vi "Append Block Diagram Image.vi"(0 "PDF Report IN":refnum<class "PDF Report Class.lvclass">, 1 "Image size":T1={"Maximum Width"=-1, "Maximum Height"=-1}, 2 "Scale (%)":sgl=100.0, 3 "Border":T2={"Show?"=FALSE, "Thickness (point)"=0.5, "Color"=0}, 5 "VI reference":refnum<vi>, 11 "error in (no error)":errorcluster, 12 "Caption":string, 14 "Position and indentation":T3={"Alignment"=enum."Center", "X "=0.0, "Y"=0.0, "Indentation"=0.0}) -> (4 "PDF Report OUT":refnum<class "PDF Report Class.lvclass">, 15 "error out":errorcluster)   [LabVIEW 2020, in "Exaprom PDF.lvlib"]
doc: "Creates an image of the block diagram of the VI you specify in <B>VI reference</B> and appends it to a PDF report. <B>Not Available in Run-Time </B>.\n\n<B>FRANÇAIS</B>\nCréation de l'image du \"block diagram\" que vous avez spécifié par <B>VI reference</B> et ajout au rapport PDF. <B>Ce VI fonctionne uniquement en mode développement</B>.\n\nVersion 1.0\nDeveloped by Jean-Marc Simard\nCopyright © 2010, Exaprom Inc.\nAll rights reserved.\nLicense: BSD\n\nWith iTextSharp 4.1.6 (http://itextsharp.sourceforge.net)\nunder Mozilla Public License Version 1.1\n(http://www.mozilla.org/MPL/MPL-1.1.html)"
uses:
  <userlib>/labview-PDF-writer-master/Exaprom PDF.lvlib
  <userlib>/labview-PDF-writer-master/LV Class/PDF Report Class/PDF Report Class.lvclass
  <userlib>/labview-PDF-writer-master/Controls/Image Controls/Image alignment and position.ctl
  <userlib>/labview-PDF-writer-master/Controls/Image Controls/Image aligment.ctl
  <userlib>/labview-PDF-writer-master/Controls/Image Controls/Image border.ctl
  <userlib>/labview-PDF-writer-master/Controls/Image Controls/Image Size Block Diagram.ctl
  <userlib>/labview-PDF-writer-master/Controls/Font Controls/Font complete cluster.ctl
  <userlib>/labview-PDF-writer-master/Controls/Font Controls/Font size.ctl
  <userlib>/labview-PDF-writer-master/Controls/Font Controls/Font color.ctl
  <userlib>/labview-PDF-writer-master/Controls/Font Controls/Type and encoding.ctl
  <userlib>/labview-PDF-writer-master/Controls/Text Controls/Unicode/Type and run direction.ctl
  C:/Program Files (x86)/National Instruments/LabVIEW 2020/user.lib/labview-PDF-writer-master/DLL/itextsharp.dll
  DLL/itextsharp.dll
panel:
  out "Size (points)":cluster{"TotalHeight":sgl, "TotalWidth":sgl}
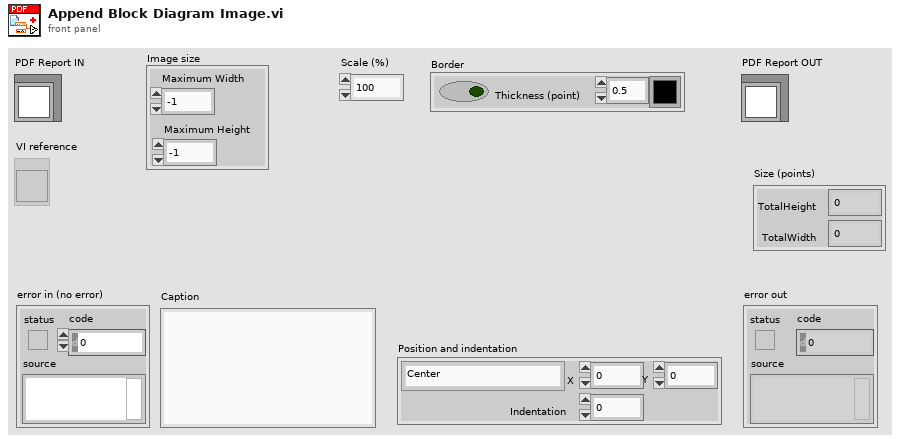
[diagram p1: front panel]
types:
  T1 = typedef "Exaprom PDF.lvlib/Image Size Block Diagram.ctl" = cluster{"Maximum Width":i32, "Maximum Height":i32}
  T2 = typedef "Exaprom PDF.lvlib/Image border.ctl" = cluster{"Show?":bool, "Thickness (point)":sgl, "Color":u32}
  T3 = typedef "Exaprom PDF.lvlib/Image alignment and position.ctl" = cluster{"Alignment":T4, "X ":sgl, "Y":sgl, "Indentation":sgl}
  T4 = typedef "Exaprom PDF.lvlib/Image aligment.ctl" = enum16{"Absolute (X,Y)", "Left", "Center", "Right", "Left (textwrap)", "Right (textwrap)"}
  T5 = typedef "Exaprom PDF.lvlib/Font complete cluster.ctl" = cluster{"Name":string, "Size":T6, "Color":T7, "Style":cluster{"Bold":bool, "Italic":bool, "Underline":bool, "Strikeout":bool}, "Type":T8}
  T6 = typedef "Exaprom PDF.lvlib/Font size.ctl" = sgl
  T7 = typedef "Exaprom PDF.lvlib/Font color.ctl" = u32
  T8 = typedef "Exaprom PDF.lvlib/Type and encoding.ctl" = cluster{"Type&direction":T9, "Embedded":bool, "Encoding":string}
  T9 = typedef "Exaprom PDF.lvlib/Type and run direction.ctl" = enum16{"Select", "ASCII", "UTF-16", "UTF-16 (default)", "UTF-16 (LTR)", "UTF-16 (RTL)"}
  T10 = enum32{"invalid app kind", "Development System", "Run Time System", "Student Edition", "Embedded LabVIEW", "Evaluation", "Custom"}
  T11 = typedef "imagedata.ctl" = cluster{"image type":i32, "image depth":i32, "image":u8[], "mask":u8[], "colors":u32[], "Rectangle":cluster{"left":i16, "top":i16, "right":i16, "bottom":i16}}
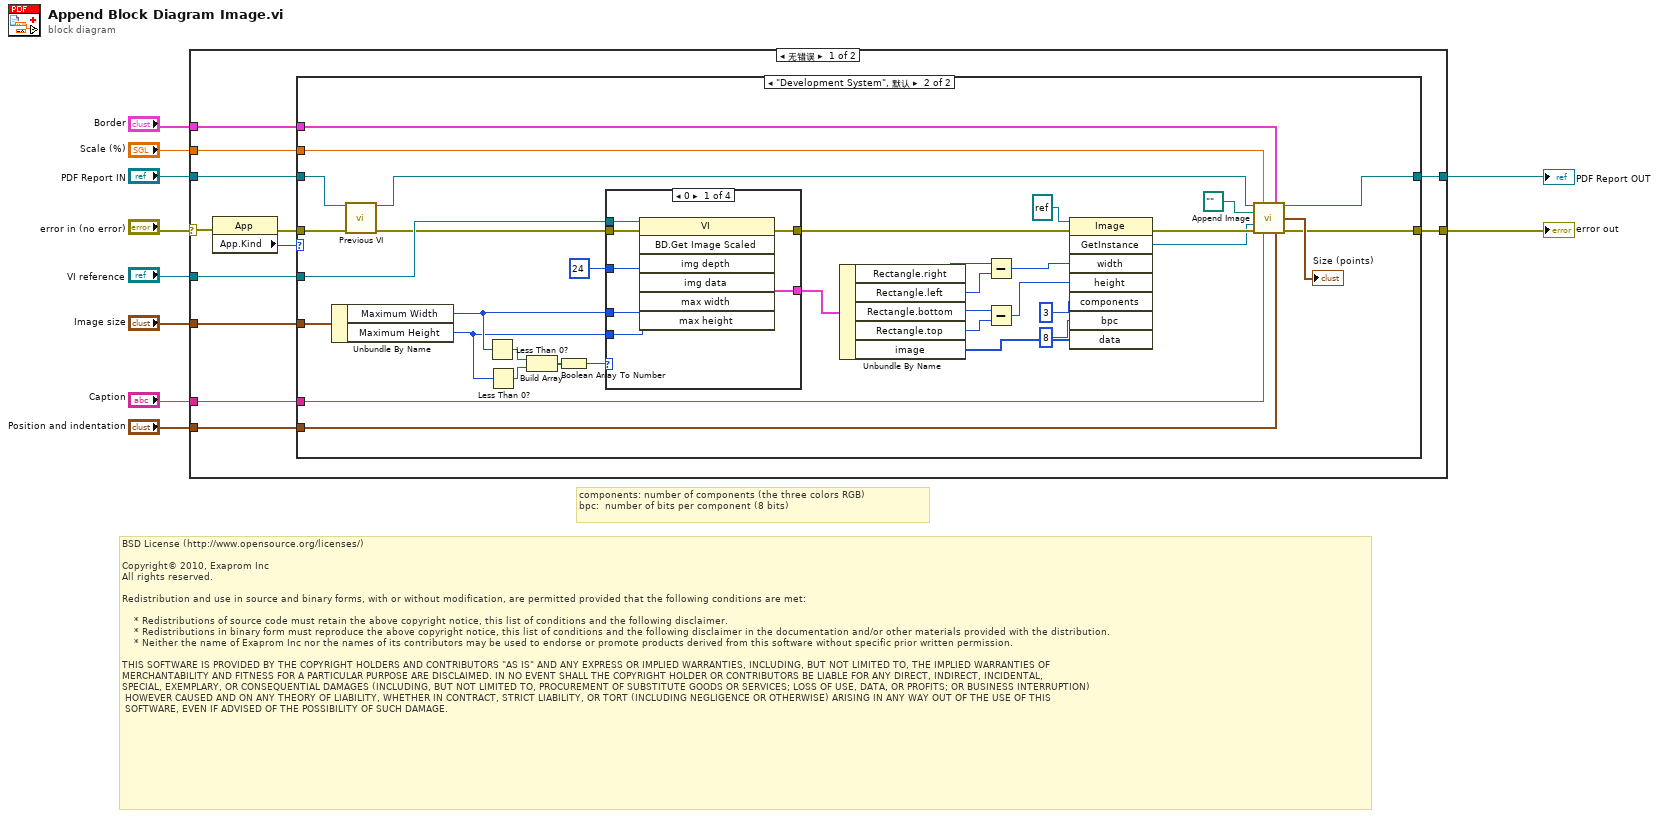
[diagram p0: block diagram]
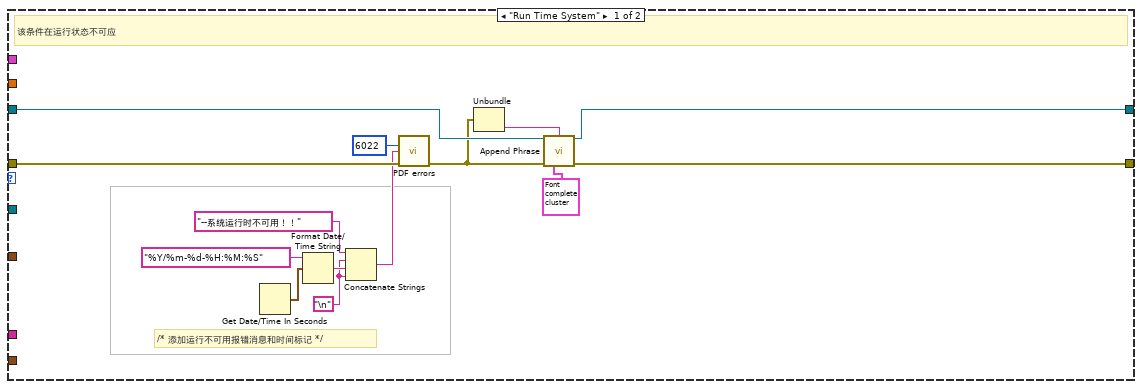
[diagram p2: hidden frame]
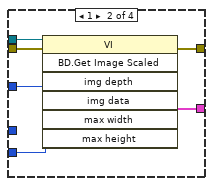
[diagram p3: hidden frame]
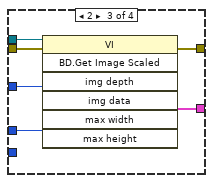
[diagram p4: hidden frame]
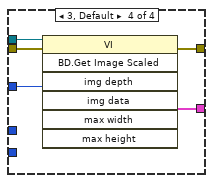
[diagram p5: hidden frame]
diagram:
  # "components: number of components (the three colors RGB)\nbpc:  number of bits per component (8 bits)"
  # "BSD License (http://www.opensource.org/licenses/)\n\nCopyright© 2010, Exaprom Inc\nAll rights reserved.\n\nRedistribution and use in source and binary forms, with or without modification, are permitted provided that the following conditions are met:\n\n    * Redistributions of source code must retain the above copyright notice, this list of conditions and the following disclaimer.\n    * Redistributions in binary form must reproduce the above copyright notice, this list of conditions and the following disclaimer in the documentation and/or other materials provided with the distribution.\n    * Neither the name of Exaprom Inc nor the names of its contributors may be used to endorse or promote products derived from this software without specific prior written permission.\n\nTHIS SOFTWARE IS PROVIDED BY THE COPYRIGHT HOLDERS AND CONTRIBUTORS \"AS IS\" AND ANY EXPRESS OR IMPLIED WARRANTIES, INCLUDING, BUT NOT LIMITED TO, THE IMPLIED WARRANTIES OF \nMERCHANTABILITY AND FITNESS FOR A PARTICULAR PURPOSE ARE DISCLAIMED. IN NO EVENT SHALL THE COPYRIGHT HOLDER OR CONTRIBUTORS BE LIABLE FOR ANY DIRECT, INDIRECT, INCIDENTAL,\nSPECIAL, EXEMPLARY, OR CONSEQUENTIAL DAMAGES (INCLUDING, BUT NOT LIMITED TO, PROCUREMENT OF SUBSTITUTE GOODS OR SERVICES; LOSS OF USE, DATA, OR PROFITS; OR BUSINESS INTERRUPTION)\n HOWEVER CAUSED AND ON ANY THEORY OF LIABILITY, WHETHER IN CONTRACT, STRICT LIABILITY, OR TORT (INCLUDING NEGLIGENCE OR OTHERWISE) ARISING IN ANY WAY OUT OF THE USE OF THIS\n SOFTWARE, EVEN IF ADVISED OF THE POSSIBILITY OF SUCH DAMAGE."
  n1 = case shown="无错误" "error in (no error)" {
    selector: "error in (no error)" -> [w11 w97]
    tunnel: [w19 w97] -> w3
    tunnel: "VI reference" -> [w22 _]
    tunnel: [w20 w96] -> w2
    tunnel: "PDF Report IN" -> [w21 w96]
    tunnel: "Caption" -> [w18 _]
    tunnel: "Position and indentation" -> [w17 _]
    tunnel: "Border" -> [w16 _]
    tunnel: "Scale (%)" -> [w15 _]
    tunnel: "Image size" -> [w14 _]
    frame No Error {
      n2 = property class="App"(error in=w11) -> (error out=w12:errorcluster, "App.Kind"=w13:T10)  [unwired: 1 in, 1 out]
      n3 = case shown="\"Development System\", 默认" w13 {
        tunnel: w22 -> [_ w71]
        tunnel: w21 -> [w34 w68]
        tunnel: [w33 w37] -> w20
        tunnel: [w32 w38] -> w19
        tunnel: w18 -> [_ w67]
        tunnel: w17 -> [_ w66]
        tunnel: w16 -> [_ w65]
        tunnel: w15 -> [_ w64]
        tunnel: w12 -> [w36 w61]
        tunnel: w14 -> [_ w59]
        frame "Run Time System" {
          w25 = "\n"
          # "/* 添加运行不可用报错消息和时间标记 */"
          # "该条件在运行状态不可应"
          n4 = Get Date/Time In Seconds() -> (seconds since 1Jan1904=w28:timestamp)
          n5 = Format Date/Time String(time format string (%c)="%Y/%m-%d-%H:%M:%S" ("时间格式字符串(%c)"), seconds (now)=w28) -> (date/time string=w27:string)  [unwired: 1 in]
          n6 = Concatenate Strings("--系统运行时不可用！！" ("Additionnal information"), w25, w27, w25) -> (w23:string)
          n7 = call <userlib>:"PDF errors.vi"("code"=6022, "Additionnal information"=w23, "error in (no error)"=w36) -> ("error out"=w31:errorcluster)  [unwired: 12 out]
          n8 = Unbundle(w31) -> ("source"=w30:string)  [unwired: 2 out]
          n9 = call <userlib>:"Append Phrase.vi"("PDF Report IN"=w34, "Text"=w30, "error in (no error)"=w31, "Font"=T5 {"Name"="", "Size"=-1.0, "Color"=16711680, "Style"={"Bold"=TRUE, "Italic"=FALSE, "Underline"=FALSE, "Strikeout"=FALSE}, "Type"={"Type&direction"=enum."Select", "Embedded"=FALSE, "Encoding"=""}} ("Font complete")) -> ("PDF Report OUT"=w33:refnum<class "PDF Report Class.lvclass">, "error out"=w32:errorcluster)  [unwired: 1 in, 9 out]
        }
        frame "Development System", Default {
          n10 = Unbundle By Name(w59) -> ("Maximum Width"=w45:i32, "Maximum Height"=w44:i32)
          n11 = call <userlib>:"Previous VI.vi"("PDF Report IN"=w68, "error in (no error)"=w61) -> ("PDF Report OUT"=w39:refnum<class "PDF Report Class.lvclass">, "error out"=w60:errorcluster)  [unwired: 12 out]
          n12 = Less Than 0?(x=w45) -> (x < 0?=w43:bool)
          n13 = Less Than 0?(x=w44) -> (x < 0?=w42:bool)
          n14 = Build Array(w43, w42) -> (w41:bool[])
          n15 = Boolean Array To Number(Boolean array=w41) -> (number=w40:u32)
          n16 = case shown="0" w40 {
            tunnel: [w78 w84 w90 w95] -> w58
            tunnel: w71 -> [w77 w83 w89 w94]
            tunnel: [w76 w82 w88 w93] -> w47
            tunnel: 24 ("Image Depth") -> [w75 w81 w87 w92]
            tunnel: w60 -> [w74 w80 w86 w91]
            tunnel: w45 -> [w73 _ w85 _]
            tunnel: w44 -> [w72 w79 _ _]
            frame 0 {
              n17 = invoke class="VI" method="BD.Get Image Scaled"(reference=w77, error in=w74, "img depth"=w75, "max width"=w73, "max height"=w72) -> (error out=w78:errorcluster, "img data"=w76:T11)  [unwired: 2 in, 5 out]
            }
            frame 1 {
              n18 = invoke class="VI" method="BD.Get Image Scaled"(reference=w83, error in=w80, "img depth"=w81, "max height"=w79) -> (error out=w84:errorcluster, "img data"=w82:T11)  [unwired: 3 in, 5 out]
            }
            frame 2 {
              n19 = invoke class="VI" method="BD.Get Image Scaled"(reference=w89, error in=w86, "img depth"=w87, "max width"=w85) -> (error out=w90:errorcluster, "img data"=w88:T11)  [unwired: 3 in, 5 out]
            }
            frame 3, Default {
              n20 = invoke class="VI" method="BD.Get Image Scaled"(reference=w94, error in=w91, "img depth"=w92) -> (error out=w95:errorcluster, "img data"=w93:T11)  [unwired: 4 in, 5 out]
            }
          }
          n21 = Unbundle By Name(w47) -> ("Rectangle.right"=w56:i16, "Rectangle.left"=w55:i16, "Rectangle.bottom"=w53:i16, "Rectangle.top"=w52:i16, "image"=w49:u8[])
          n22 = Subtract(x=w56, y=w55) -> (x-y=w54:i16)
          n23 = Subtract(x=w53, y=w52) -> (x-y=w51:i16)
          n24 = invoke class="Image" method="GetInstance"(reference=refnum<k24> refnum ("image"), error in=w58, "width"=w54, "height"=w51, "components"=3, "bpc"=8, "data"=w49) -> (error out=w69:errorcluster, "GetInstance"=w63:refnum<k24>)  [unwired: 1 in, 6 out]
          n25 = call <userlib>:"Append Image.vi"("PDF Report IN"=w39, "Scale (%)"=w64, "Border"=w65, "Image path"=path "" ("path"), "Image Ref iTexSharp"=w63, "error in (no error)"=w69, "Caption"=w67, "Position and indentation"=w66) -> ("PDF Report OUT"=w37:refnum<class "PDF Report Class.lvclass">, "Size (points)"=→"Size (points)":cluster{"TotalHeight":sgl, "TotalWidth":sgl}, "error out"=w38:errorcluster)  [unwired: 5 out]
        }
      }
    }
    frame Error {
    }
  }
  "error out" <- w3
  "PDF Report OUT" <- w2
